vi "TestProgram.vi"() -> ()   [LabVIEW 2011]
uses:
  <instrlib>/Newport ESP301/Newport ESP301.lvlib
panel:
  out "StrehlRatio":dbl=nan
  out "error (scalar)":dbl=nan
  out "Image (IMAQ)":T1(plugin-control)
  in  "Save":bool
  in  "Info":string
  in  "folder":path
  in  "clear daTA":bool
  out "new picture":picture
  out "standard deviation total":dbl=-0.0 format="%0.2f"
  in  "file name":string
  out "Waveform Graph":dbl[][](graph)
  in  "setVelo":dbl=20.0
  in  "cONTINIOUS":bool
  in  "collect daTA":bool
  out "Array":dbl[][](array[numeric])
  out "Value 2":dbl(graph)
  out "Value":dbl(graph)
  out "centroidy":dbl
  out "acceleration":dbl(graph)
  in  "time to wait (TCP) 2":i32=10
  out "Data String":string
  out "shot number":i32=65426
  in  "Device Name":string="StagingFocusBeam2"
  out "centroidx":dbl
  out "Remote Host":string="192.168.10.115"
  out "port or service name":u16=65418
  out "x-y":dbl(knob) scale=0.0..100.0
  out "error out 4":errorcluster
  in  "sTEPsIZE":dbl=5.0
  out "Position (units) 2":dbl(graph)=-13324.641
  in  "ScaN":bool
  in  "shake":bool
  in  "Cluster":T2={"increase"=0.004, "min velocity"=0.1, "max velocity"=3.0, "Stop increase"=0.02}
  out "appended array":dbl[][](graph)=[[1.0, 0.7046880791959296, 0.4965852858533471, 0.3499377259476329, 0.2465969370957652, 0.1737739140097176, 0.12245639698366893, 0.08629355394147512, 0.06081002915927391, 0.0628100291592739, 0.0648100291592739, 0.0668100291592739, 0.06881002915927391, 0.08881002915927391, 0.12881002915927392, 0.18881002915927392, 0.26881002915927393, 0.36881002915927397, 0.48881002915927396, 0.628810029159274, 0.788810029159274, 0.968810029159274, 1.0], [0.0, 0.0, 0.0, 0.0, 0.0, 0.0, 0.004000000000814907, 0.002999999998792191, 0.040000000000873115, 0.20499999999992724, 0.363999999999578, 0.5879999999997381, 0.7160000000003492, 0.7360000000007858, 0.7879999999986467, 0.6760000000012951, 0.3989999999994325, 0.01300000000082946, 0.004000000000814907, 0.003999999998995918, 0.0, 0.0, 0.0], [0.0, 0.0, 0.0, 0.0, 0.0, 0.0, 0.004000000000814907, -0.0010000000020227162, 0.037000000002080924, 0.16499999999905413, 0.15899999999965075, 0.22400000000016007, 0.12800000000061118, 0.020000000000436557, 0.05199999999786087, -0.11199999999735155, -0.27700000000186265, -0.385999999998603, -0.009000000000014552, -1.8189894035458565e-12, -0.003999999998995918, 0.0, 0.0]]
  out "error out 3":errorcluster
  out "ratio":dbl(graph)=1.0
  out "velocity":dbl(graph)
  in  "Velocity (units/s) 2":dbl
  in  "RedRatio":dbl=1.0
  in  "Step":bool
  out "Reduction Ratio":dbl format="%.6g"
  out "Power Status":bool=TRUE
  out "Velocity (units/s)":dbl format="%.4g"
  out "Position (units)":dbl(graph)=-13329.169
  in  "Axis (1)":i32=2
  out "error out":errorcluster
  in  "stop":bool
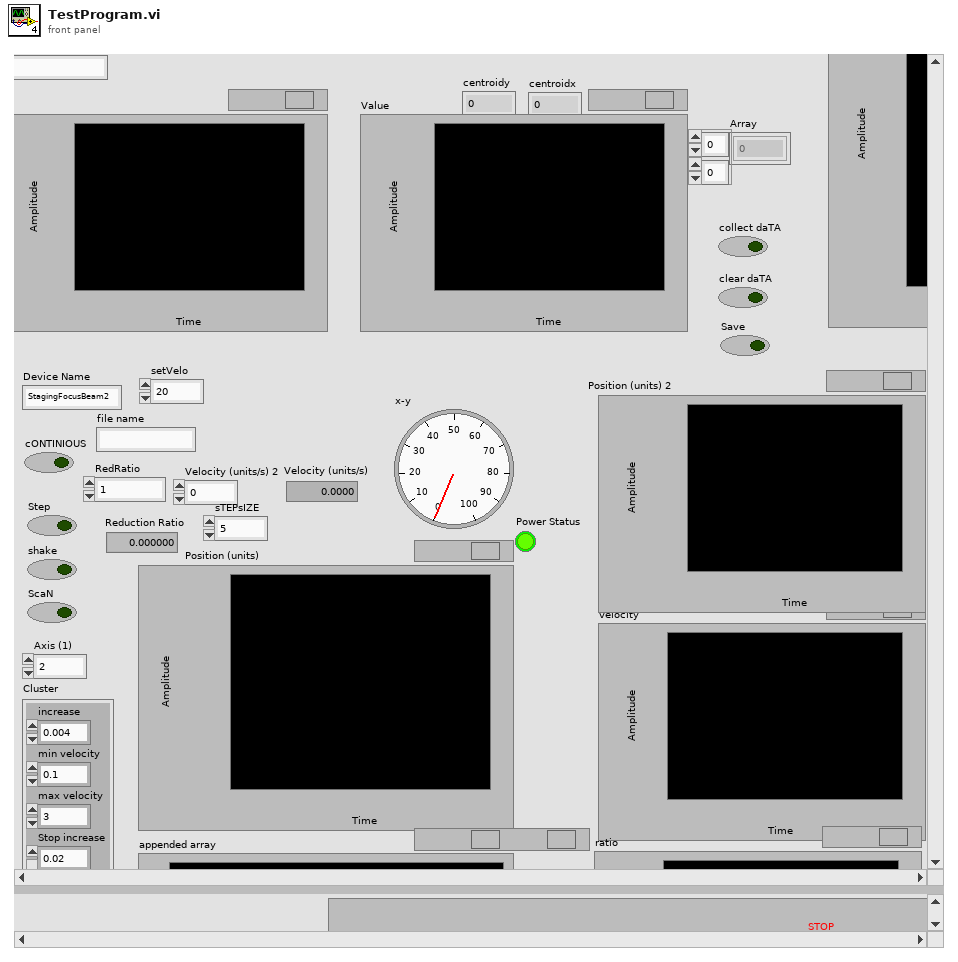
[diagram p1: front panel]
types:
  T1 = typedef "IMAQ Image.ctl" = refnum<image>
  T2 = cluster{"increase":dbl, "min velocity":dbl, "max velocity":dbl, "Stop increase":dbl}
  T3 = typedef "Image Type" = u32
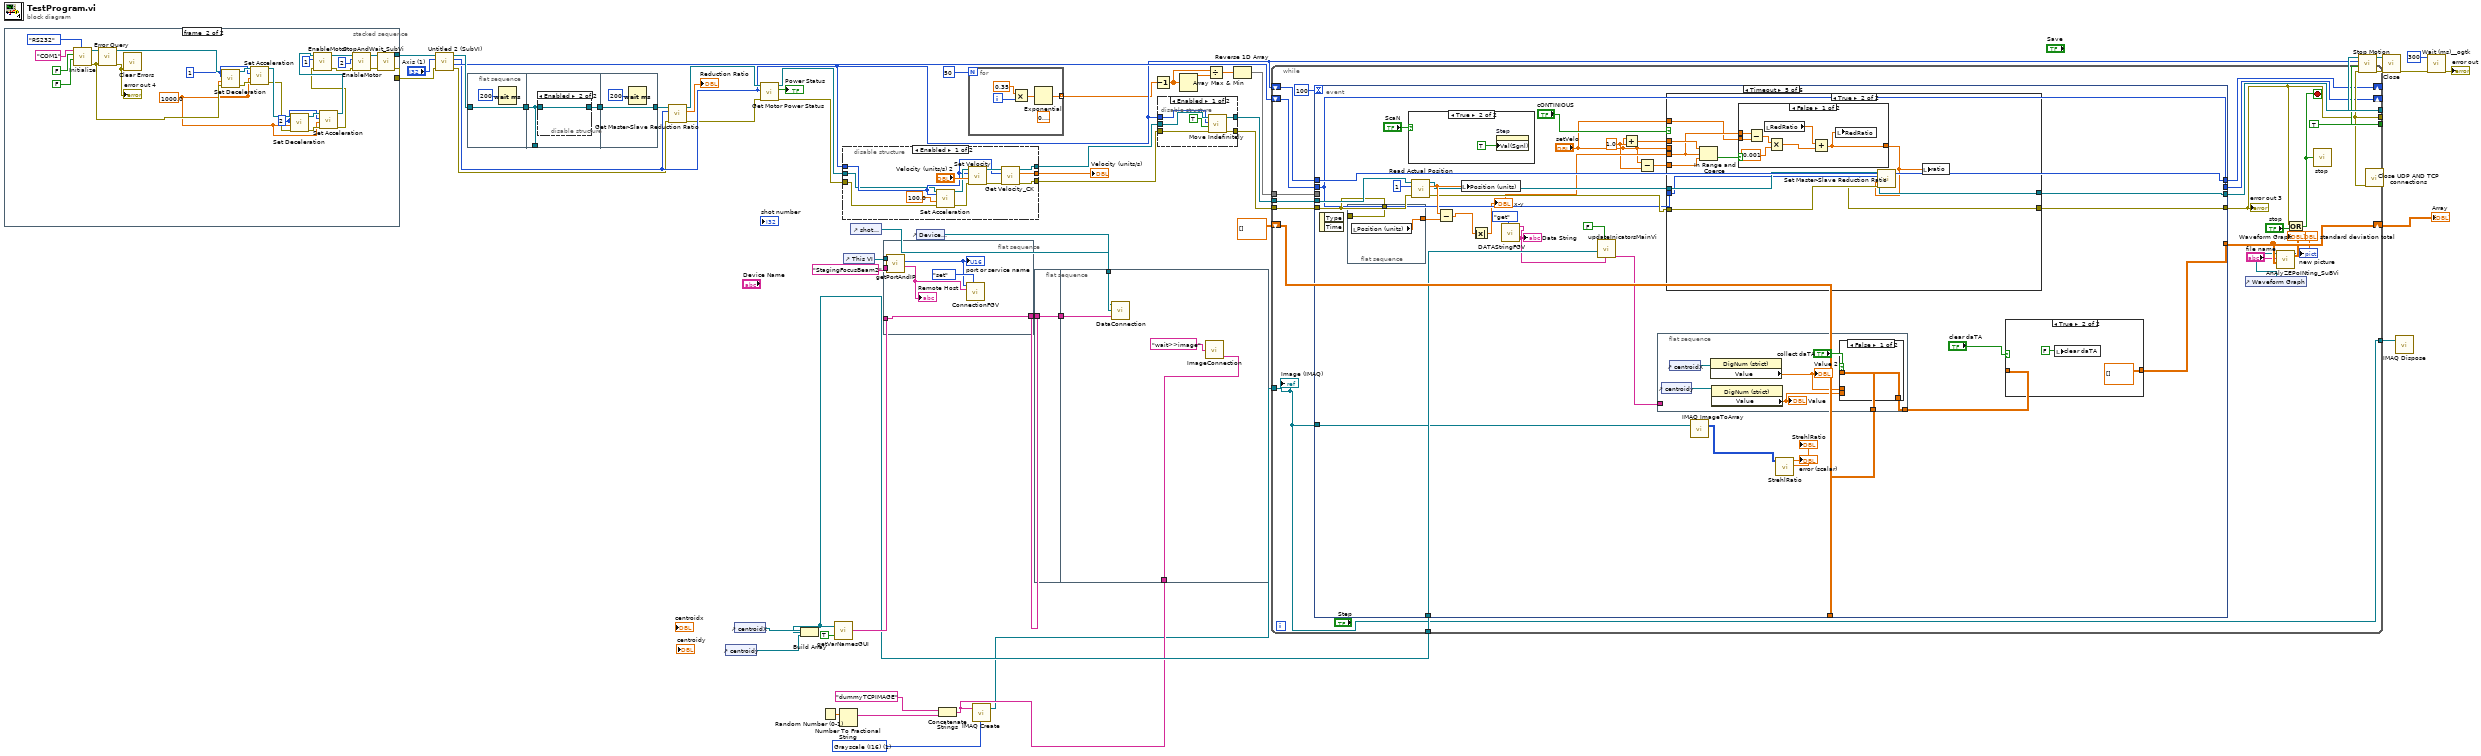
[diagram p0: block diagram]
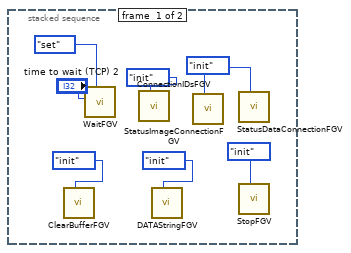
[diagram p2: hidden frame]
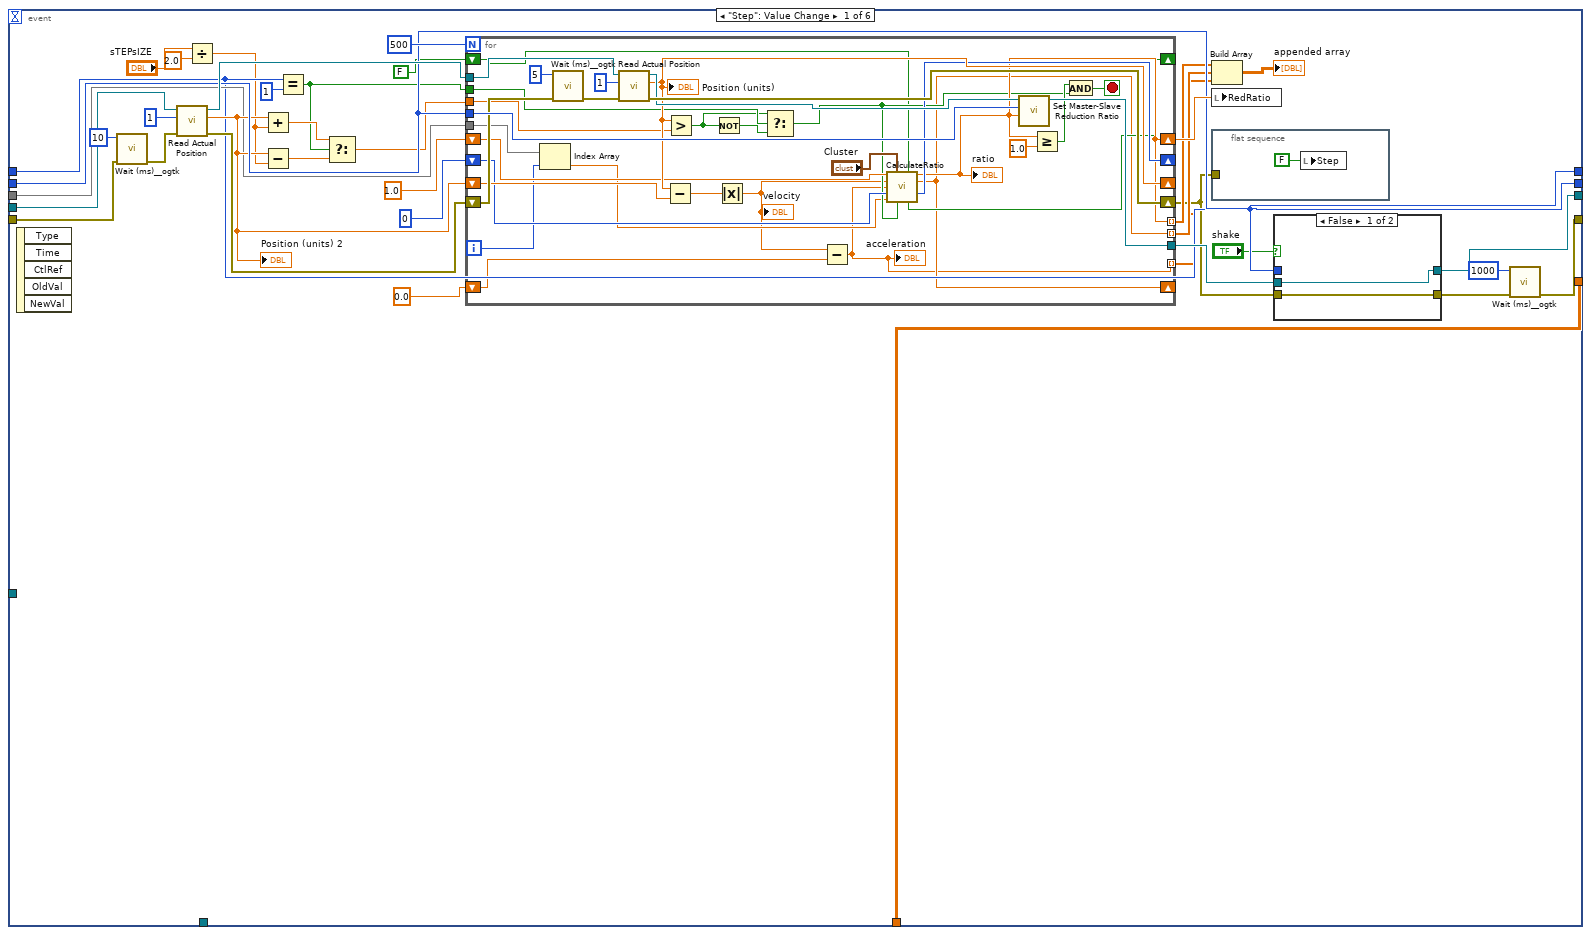
[diagram p3: hidden frame]
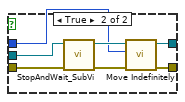
[diagram p4: hidden frame]
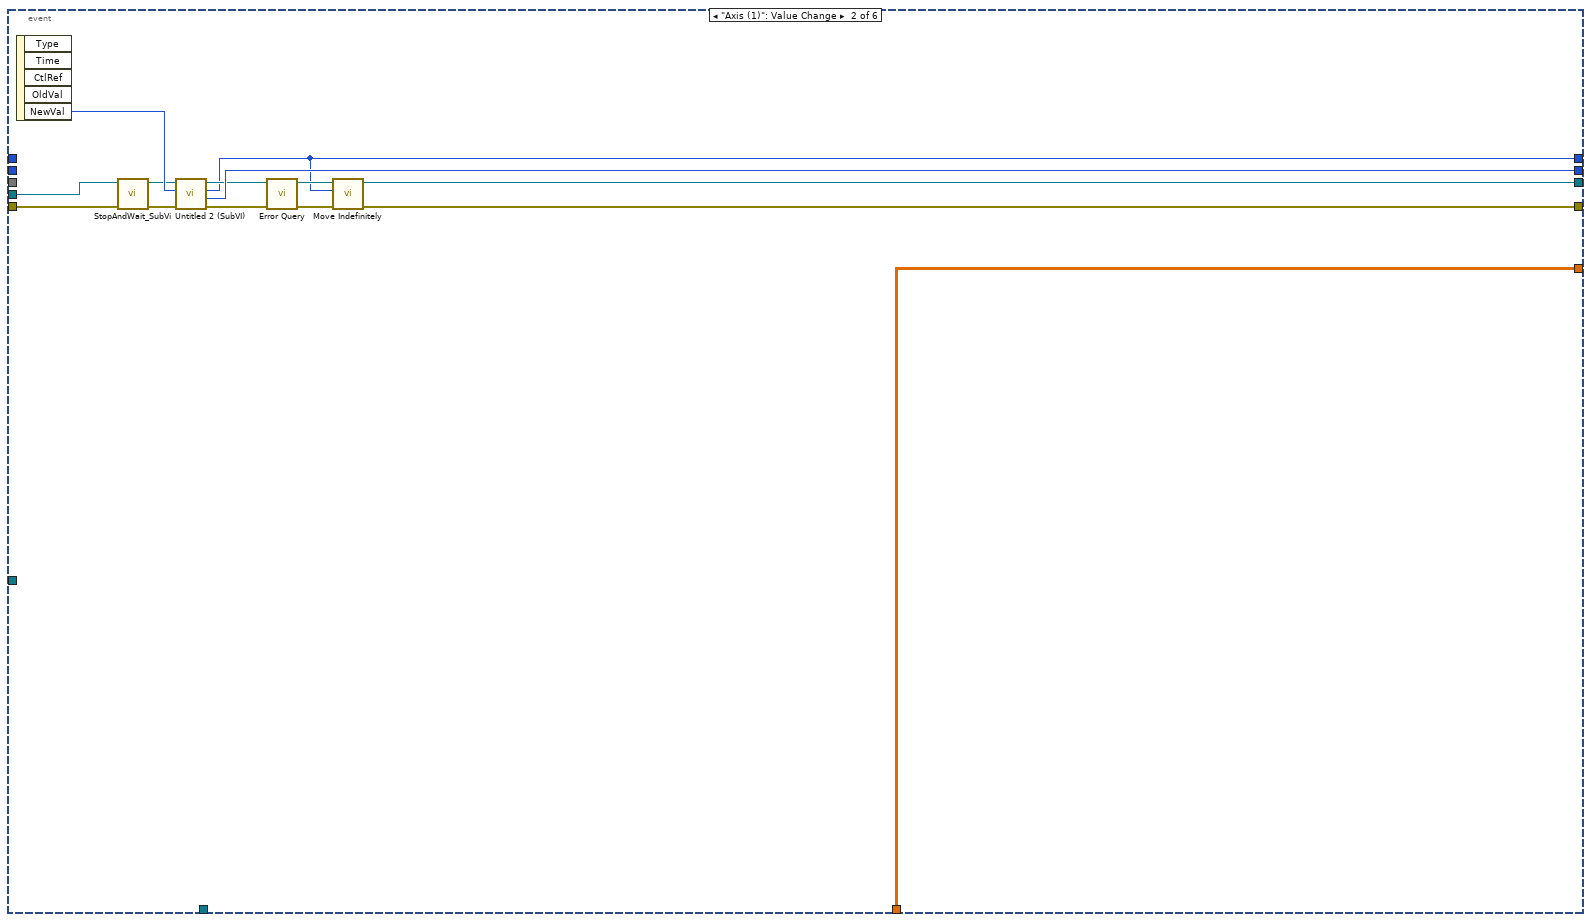
[diagram p5: hidden frame]
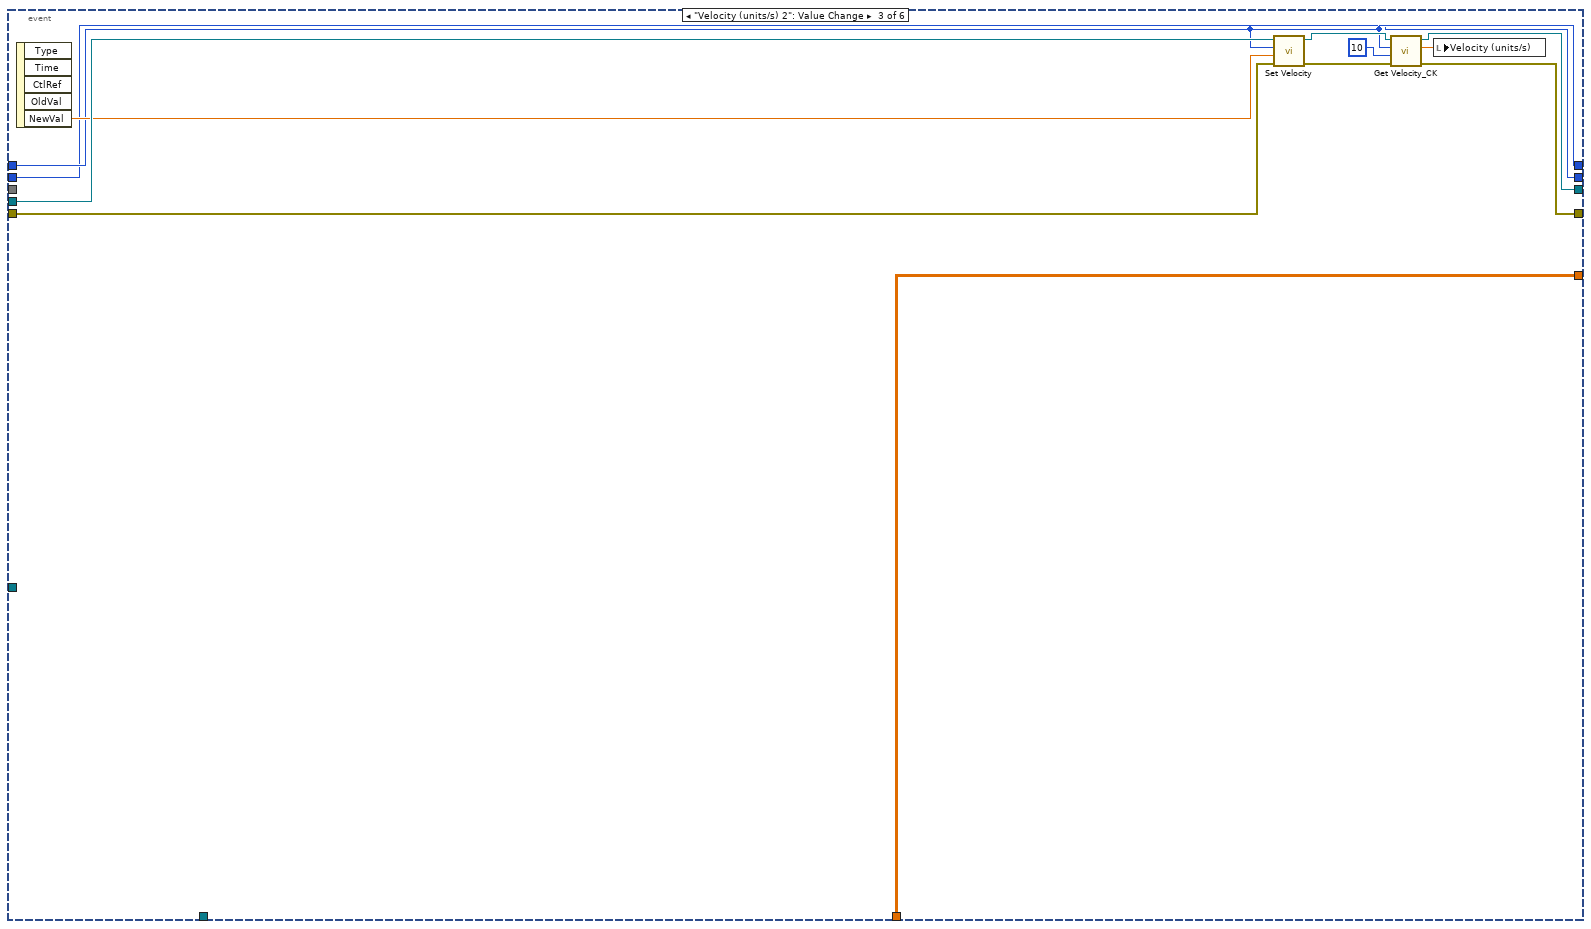
[diagram p6: hidden frame]
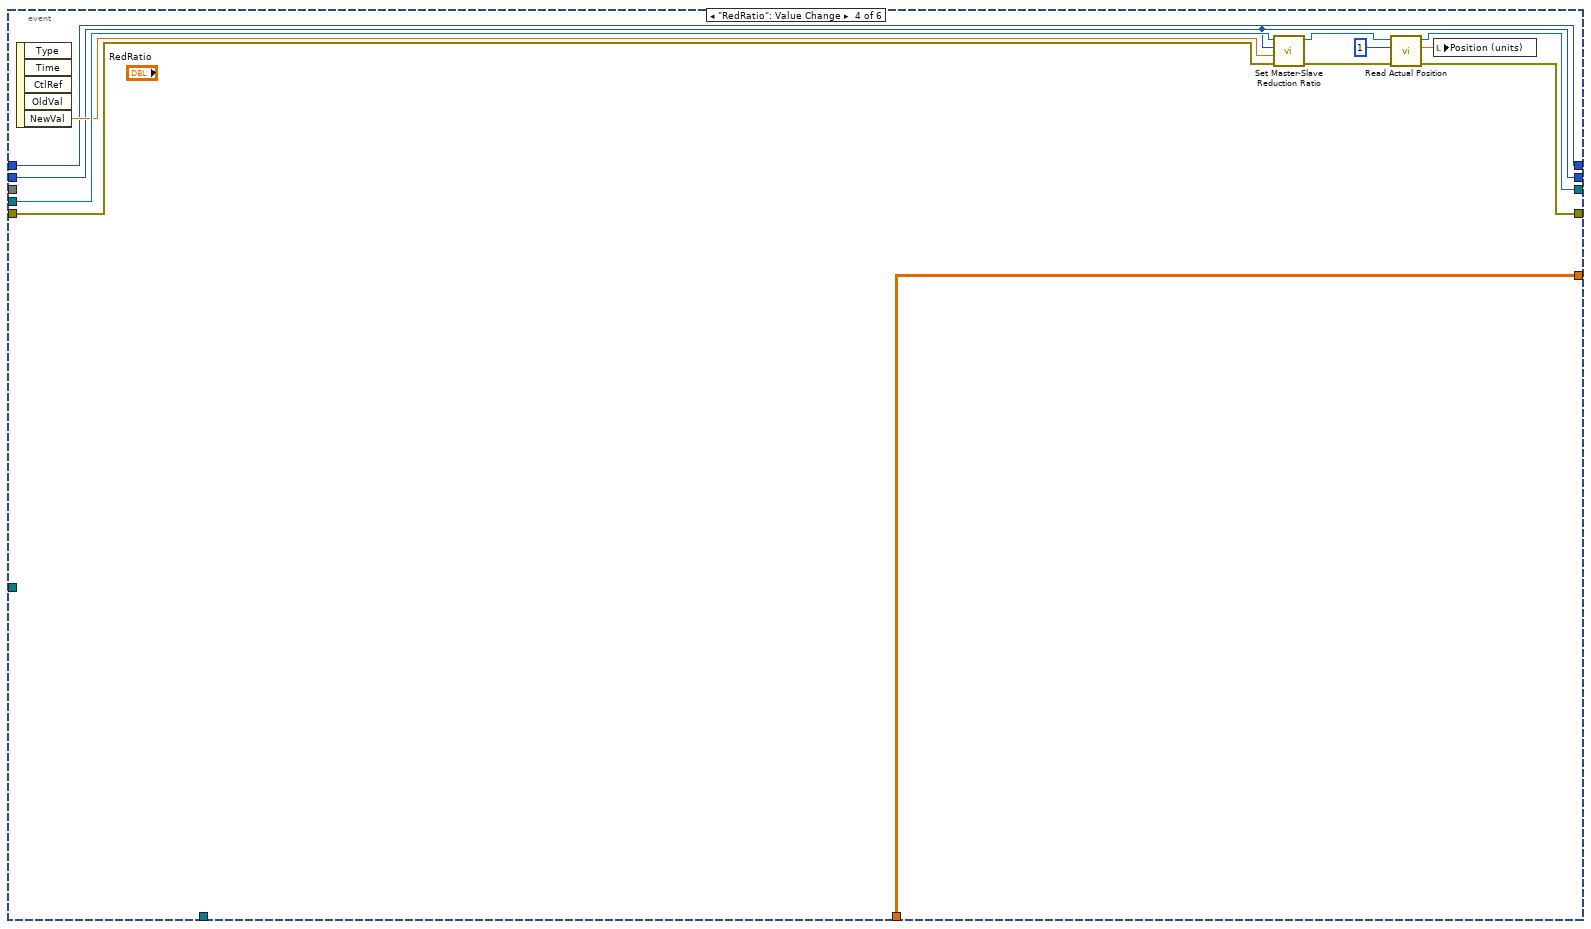
[diagram p7: hidden frame]
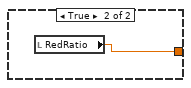
[diagram p10: hidden frame]
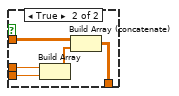
[diagram p11: hidden frame]
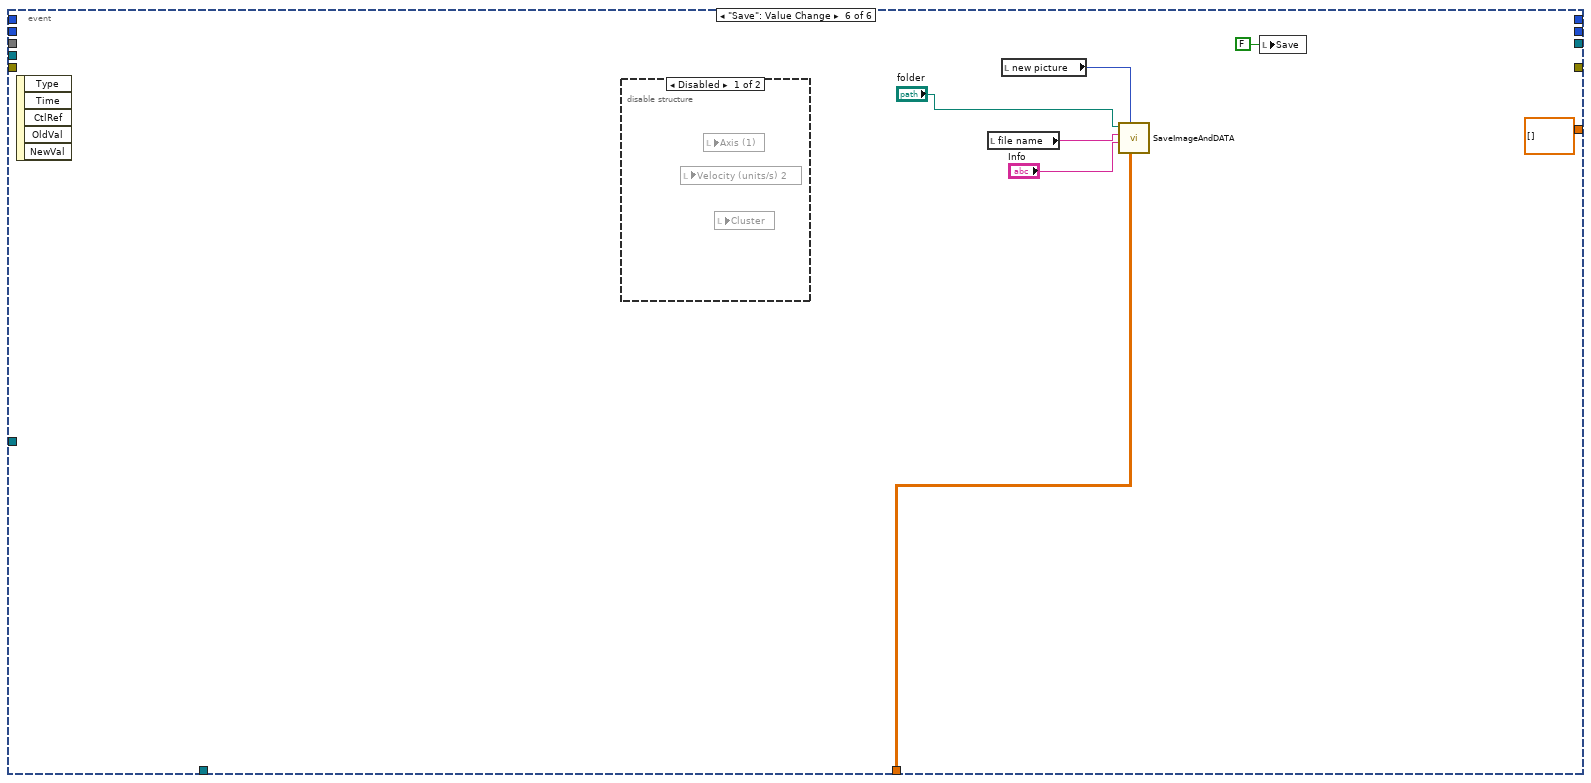
[diagram p13: hidden frame]
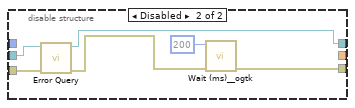
[diagram p15: hidden frame]
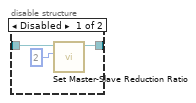
[diagram p16: hidden frame]
diagram:
  w3 = T3 1 items=["Grayscale (U8)", "Grayscale (I16)", "Grayscale (SGL)", "Complex (CSG)", "RGB (U32)", "HSL (U32)", "RGB (U64)", "Grayscale (U16)"] ("Image Type")
  n1 = stacked-sequence {
    tunnel: [_ w85] -> w23
    tunnel: [_ w84] -> w22
    frame #0 {
      w59 = enum16{"get", "set", "init"}."init" ("Command")
      n2 = call "ClearBufferFGV.vi"("Command"=enum16{"set", "get", "init"}."init") -> ()  [unwired: 10 in, 1 out]
      n3 = call "WaitFGV.vi"("Command"=enum16{"get", "set", "init"}."set", "milliseconds to wait"="time to wait (TCP) 2") -> ()  [unwired: 9 in, 1 out]
      n4 = call "ConnectionIDsFGV.vi"("Command"=enum16{"add", "get", "init"}."init") -> ()  [unwired: 10 in, 1 out]
      n5 = call "DATAStringFGV.vi"("Command"=enum16{"get", "set", "init"}."init") -> ()  [unwired: 10 in, 1 out]
      n6 = call "StatusImageConnectionFGV.vi"("Command"=w59) -> ()  [unwired: 10 in, 1 out]
      n7 = call "StatusDataConnectionFGV.vi"("Command"=w59) -> ()  [unwired: 10 in, 1 out]
      n8 = call "StopFGV.vi"("Command"=enum16{"set", "get", "init"}."init") -> ()  [unwired: 10 in, 1 out]
    }
    frame #1 {
      w63 = 2 ("Axis (1)")
      w71 = 1 ("Axis (1) 2")
      w64 = 1000.0 ("Acceleration (0 units/s²)")
      n9 = call <instrlib>:"Initialize.vi"("VISA resource name"="COM1" ("Settings.devport"), "ID Query (True)"=FALSE, "Reset (False)"=FALSE, "Serial Link (RS232)"=enum16{"RS232", "USB"}."RS232") -> ("VISA resource name out"=w83:refnum<visa-resource-name>, "error out"=w73:errorcluster)  [unwired: 5 in]
      n10 = call <instrlib>:"Error Query.vi"("error in (no error)"=w73, "VISA resource name"=w83) -> ("error out"=w82:errorcluster, "VISA resource name out"=w75:refnum<visa-resource-name>)  [unwired: 2 in, 2 out]
      "error out 4" <- w82
      n11 = call <vilib>:"Clear Errors.vi"("error in (no error)"=w82) -> ()  [unwired: 6 in, 1 out]
      n12 = call <instrlib>:"Set Deceleration.vi"("error in (no error)"=w73, "Deceleration (0 units/s²)"=w64, "Axis (1)"=w71, "VISA resource name"=w75) -> ("error out"=w72:errorcluster, "VISA resource name out"=w74:refnum<visa-resource-name>)  [unwired: 2 in]
      n13 = call <instrlib>:"Set Acceleration.vi"("error in (no error)"=w72, "Acceleration (0 units/s²)"=w64, "Axis (1)"=w71, "VISA resource name"=w74) -> ("error out"=w66:errorcluster, "VISA resource name out"=w68:refnum<visa-resource-name>)  [unwired: 2 in]
      n14 = call <instrlib>:"Set Deceleration.vi"("error in (no error)"=w66, "Deceleration (0 units/s²)"=w64, "Axis (1)"=w63, "VISA resource name"=w68) -> ("error out"=w70:errorcluster, "VISA resource name out"=w69:refnum<visa-resource-name>)  [unwired: 2 in]
      n15 = call <instrlib>:"Set Acceleration.vi"("error in (no error)"=w70, "Acceleration (0 units/s²)"=w64, "Axis (1)"=w63, "VISA resource name"=w69) -> ("error out"=w65:errorcluster, "VISA resource name out"=w67:refnum<visa-resource-name>)  [unwired: 2 in]
      n16 = call "EnableMotor.vi"("error in (no error)"=w65, "Axis (1) in"=1, "VISA Refnum in"=w67) -> ("error out"=w79:errorcluster, "VISA Refnum out"=w77:refnum<visa-resource-name>)  [unwired: 7 in]
      n17 = call "EnableMotor.vi"("error in (no error)"=w79, "Axis (1) in"=2, "VISA Refnum in"=w77) -> ("error out"=w78:errorcluster, "VISA Refnum out"=w76:refnum<visa-resource-name>)  [unwired: 7 in]
      n18 = call "StopAndWait_SubVi.vi"("error in (no error)"=w78, "VISA Refnum in"=w76) -> ("error out"=w84:errorcluster, "VISA Refnum out"=w85:refnum<visa-resource-name>)  [unwired: 8 in]
    }
  }
  n19 = call "Untitled 2 (SubVI).vi"("error in (no error)"=w22, "Axis (1)"="Axis (1)", "VISA Refnum in"=w23) -> ("error out"=w26:errorcluster, "Slave"=w35:i32, "Master"=w33:i32, "VISA Refnum out"=w39:refnum<visa-resource-name>)  [unwired: 5 in]
  n20 = flat-sequence {
    tunnel: w39 -> [w91]
    tunnel: [w91] -> w47
    tunnel: [w92] -> _
    tunnel: [w93] -> w48
    tunnel: w47 -> [w92]
    tunnel: [w99] -> w36
    tunnel: w48 -> [w99]
    frame #0 {
      n21 = Wait (ms)(milliseconds to wait=u32 200) -> ()  [unwired: 1 out]
    }
    frame #1 {
      n22 = disable-structure shown="Enabled" {
        disable-tunnel: [w96 w97] -> w93
        disable-tunnel: w92 -> [w94 w97]
        frame Disabled {
          n23 = call <instrlib>:"Set Master-Slave Reduction Ratio.vi"("Axis (1)"=2, "VISA resource name"=w94) -> ("VISA resource name out"=w96:refnum<visa-resource-name>)  [unwired: 4 in, 1 out]
        }
        frame Enabled {
        }
      }
    }
    frame #2 {
      n24 = Wait (ms)(milliseconds to wait=u32 200) -> ()  [unwired: 1 out]
    }
  }
  n25 = call <instrlib>:"Get Master-Slave Reduction Ratio.vi"("error in (no error)"=w26, "Axis (1)"=w33, "VISA resource name"=w36) -> ("error out"=w25:errorcluster, "Reduction Ratio"=→"Reduction Ratio":dbl, "VISA resource name out"=w38:refnum<visa-resource-name>)  [unwired: 2 in]
  n26 = control-ref of="centroidy"() -> (w10:refnum<vi>)
  n27 = control-ref of="centroidX"() -> (w19:refnum<vi>)
  n28 = call <instrlib>:"Get Motor Power Status.vi"("error in (no error)"=w25, "Axis (1)"=w33, "VISA resource name"=w38) -> ("error out"=w24:errorcluster, "Power Status"=→"Power Status":bool, "VISA resource name out"=w44:refnum<visa-resource-name>)  [unwired: 2 in]
  n29 = Build Array(w19, w10) -> (w12:refnum<vi>[])
  n30 = Random Number (0-1)() -> (number: 0 to 1=w4:dbl)
  n31 = call "getVarNamesGUI.vi"("start"=TRUE, "Array"=w12) -> ("String"=w14:string)
  n32 = Number To Fractional String(number=w4) -> (F-format string=w5:string)  [unwired: 3 in]
  n33 = disable-structure shown="Enabled" {
    disable-tunnel: [w111 _] -> w55
    disable-tunnel: [w110 w116] -> w54
    disable-tunnel: w33 -> [w106 _]
    disable-tunnel: w44 -> [w104 w117]
    disable-tunnel: [w100 w113] -> w46
    disable-tunnel: w24 -> [w103 w112]
    frame Enabled {
      n34 = call <instrlib>:"Set Acceleration.vi"("error in (no error)"=w103, "Acceleration (0 units/s²)"=100.0, "Axis (1)"=w106, "VISA resource name"=w104) -> ("error out"=w102:errorcluster, "VISA resource name out"=w107:refnum<visa-resource-name>)  [unwired: 2 in]
      n35 = call <instrlib>:"Set Velocity.vi"("error in (no error)"=w102, "Velocity (units/s)"="Velocity (units/s) 2", "Axis (1)"=w106, "VISA resource name"=w107) -> ("error out"=w101:errorcluster, "VISA resource name out"=w109:refnum<visa-resource-name>)  [unwired: 2 in]
      n36 = call "Get Velocity_CK.vi"("error in (no error)"=w101, "Axis (1)"=w106, "VISA resource name"=w109) -> ("error out"=w100:errorcluster, "Velocity (units/s)"=w111:dbl, "VISA resource name out"=w110:refnum<visa-resource-name>)  [unwired: 2 in]
    }
    frame Disabled {
      n37 = call <instrlib>:"Error Query.vi"("error in (no error)"=w112, "VISA resource name"=w117) -> ("error out"=w115:errorcluster, "VISA resource name out"=w116:refnum<visa-resource-name>)  [unwired: 4 out]
      n38 = call <userlib>:"Wait (ms)__ogtk.vi"("error in (no error)"=w115, "milliseconds to wait"=u32 200) -> ("error out"=w113:errorcluster)  [unwired: 8 in, 1 out]
    }
  }
  "Velocity (units/s)" <- w55
  n39 = control-ref of="This VI"() -> (w21:refnum<vi>)
  n40 = control-ref of="shot number"() -> (w16:refnum<vi>)
  n41 = flat-sequence {
    tunnel: w21 -> [w123]
    tunnel: "StagingFocusBeam2" ("Device Name") -> [w119]
    tunnel: w14 -> [w118]
    tunnel: [w118] -> w13
    frame #0 {
      n42 = call "getPortAndIP.vi"("This Vi"=w123, "Device Name"=w119) -> ("port or service name"=w120:u16, "Remote Host"=w121:string)  [unwired: 1 in, 1 out]
      "port or service name" <- w120
      "Remote Host" <- w121
      n43 = call "ConnectionFGV.vi"("command"=enum16{"get", "set", "init"}."set", "Remote Host in"=w121, "port or service name in"=w120) -> ()  [unwired: 7 in, 2 out]
    }
  }
  n44 = control-ref of="Device Name"() -> (w17:refnum<vi>)
  n45 = Concatenate Strings("dummyTCPIMAGE" ("Image Name"), w5) -> (w2:string)
  n46 = for {
    N: 50 -> [_]
    tunnel: [w127] -> w29 mode=indexing
    i -> [w126]
    (unwired) 0.30000000000000004 ("x")
    n47 = Multiply(x=0.35, y=w126) -> (x*y=w124:dbl)
    n48 = Exponential(1:w124) -> (0:w127:dbl)
  }
  n49 = call "IMAQ Create"("Image Name"=w2, "Image Type"=w3) -> ("New Image"=w1:T1)  [unwired: 3 in, 1 out]
  n50 = flat-sequence {
    tunnel: w13 -> [w128]
    tunnel: [w128] -> w15
    tunnel: w17 -> [w132]
    tunnel: w16 -> [w131]
    tunnel: w15 -> [w133]
    tunnel: w2 -> [w129]
    frame #0 {
    }
    frame #1 {
      n51 = call "DataConnection.vi"("Subscriber list"=w133, "Device Name (h)"=w132, "shotnumber"=w131) -> ()
      n52 = call "ImageConnection.vi"("Image Name"=w129, "Image Subscriber list"="wait>>image") -> ()  [unwired: 2 in]
    }
  }
  n53 = Decrement(x=w29) -> (x-1=w30:dbl[])
  n54 = disable-structure shown="Enabled" {
    disable-tunnel: w54 -> [w139 w140]
    disable-tunnel: [w137 w140] -> w53
    disable-tunnel: w33 -> [w136 _]
    disable-tunnel: w46 -> [w135 _]
    disable-tunnel: [w134 _] -> w45
    frame Enabled {
      n55 = call <instrlib>:"Move Indefinitely.vi"("error in (no error)"=w135, "Move Direction (+)"=TRUE, "Axis (1)"=w136, "VISA resource name"=w139) -> ("error out"=w134:errorcluster, "VISA resource name out"=w137:refnum<visa-resource-name>)  [unwired: 2 in]
    }
    frame Disabled {
    }
  }
  n56 = Array Max & Min(array=w30) -> (max value=w31:dbl)  [unwired: 3 out]
  n57 = Divide(x=w30, y=w31) -> (x/y=w32:dbl[])
  n58 = Reverse 1D Array(array=w32) -> (reversed array=w27:dbl[])
  n59 = while {
    tunnel: w53 -> [w162]
    tunnel: [w161] -> w52
    tunnel: [w156] -> w11
    tunnel: [TRUE ("Stop all axes (F)")] -> w50
    tunnel: w45 -> [w159]
    shift-right: [w153] -> _
    shift-left: w33 -> [w154]
    shift-right: [w152] -> _
    shift-left: w35 -> [w158]
    tunnel: w27 -> [w151]
    tunnel: w12 -> [w150]
    shift-right: [w147] -> w8
    shift-left: dbl[][] [] -> [w148]
    tunnel: w1 -> [w141]
    tunnel: [w141] -> w7
    stop <- w149 stop-if-true
    n60 = event shown="[4] Timeout" {
      selector: _ -> [_ _ _ _ _ _]
      dyn-events: _ -> [_ _ _ _ _ _]
      timeout: 100 -> [_ _ _ _ _ _]
      tunnel: w162 -> [w199 w248 w269 w281 w313 _]
      tunnel: [w179 w249 w265 w275 w297 _] -> w161
      tunnel: w159 -> [w169 w246 w267 w279 w307 _]
      tunnel: w158 -> [w192 _ w259 w271 w294 _]
      tunnel: [w174 w250 w262 w273 w295 _] -> w156
      tunnel: w154 -> [w178 _ w260 w272 w311 _]
      tunnel: [w178 w252 w260 w272 w311 _] -> w153
      tunnel: [w192 w256 w259 w271 w294 _] -> w152
      tunnel: w151 -> [w181 _ _ _ _ _]
      tunnel: w150 -> [_ _ _ _ w305 _]
      tunnel: [w163 w244 w258 w270 w286 dbl[][] []] -> w147
      tunnel: w148 -> [w163 w244 w258 w270 w300 w358]
      tunnel: w141 -> [_ _ _ _ w285 _]
      event "Step": Value Change {
        n61 = event-data() -> ()  [unwired: 1 in, 5 out]
        n62 = call <userlib>:"Wait (ms)__ogtk.vi"("error in (no error)"=w169, "milliseconds to wait"=u32 10) -> ("error out"=w168:errorcluster)  [unwired: 8 in, 1 out]
        n63 = call <instrlib>:"Read Actual Position.vi"("error in (no error)"=w168, "Axis (1)"=1, "VISA resource name"=w199) -> ("error out"=w196:errorcluster, "Position (units)"=w189:dbl, "VISA resource name out"=w198:refnum<visa-resource-name>)  [unwired: 2 in]
        "Position (units) 2" <- w189
        n64 = Divide(x="sTEPsIZE", y=2.0) -> (x/y=w170:dbl)
        n65 = Add(x=w189, y=w170) -> (x+y=w190:dbl)
        n66 = Subtract(x=w189, y=w170) -> (x-y=w188:dbl)
        n67 = Equal?(x=w178, y=1) -> (x = y?=w186:bool)
        n68 = Select(t=w190, s=w186, f=w188) -> (s? t:f=w187:dbl)
        n69 = for {
          N: 500 -> [_]
          tunnel: [w239] -> w180
          tunnel: w198 -> [w241]
          shift-right: [w242] -> w176
          shift-left: w196 -> [w237]
          tunnel: w192 -> [w238]
          shift-right: [w232] -> _
          shift-left: w189 -> [w234]
          shift-right: [w224] -> w193
          shift-left: 1.0 -> [w223]
          tunnel: w187 -> [w231]
          tunnel: w186 -> [w229]
          shift-right: [w225] -> _
          shift-left: 0 -> [w226]
          tunnel: [w224] -> w184 mode=indexing
          tunnel: [w211] -> w183 mode=indexing
          tunnel: w181 -> [w216]
          shift-right: [w217] -> _
          shift-left: FALSE -> [w218]
          shift-right: [w211] -> _
          shift-left: 0.0 -> [w212]
          tunnel: [w210] -> w164 mode=indexing
          i -> [w215]
          stop <- w219 stop-if-true
          n70 = Index Array(array=w216, index=w215) -> (element=w214:dbl)
          n71 = call <userlib>:"Wait (ms)__ogtk.vi"("error in (no error)"=w237, "milliseconds to wait"=u32 5) -> ("error out"=w236:errorcluster)  [unwired: 8 in, 1 out]
          n72 = call <instrlib>:"Read Actual Position.vi"("error in (no error)"=w236, "Axis (1)"=1, "VISA resource name"=w241) -> ("error out"=w242:errorcluster, "Position (units)"=w232:dbl, "VISA resource name out"=w240:refnum<visa-resource-name>)  [unwired: 2 in]
          "Position (units)" <- w232
          n73 = Subtract(x=w232, y=w234) -> (x-y=w233:dbl)
          n74 = Greater?(x=w232, y=w231) -> (0:w227:bool)
          n75 = Not(x=w227) -> (.not. x?=w228:bool)
          n76 = Absolute Value(x=w233) -> (abs(x)=w213:dbl)
          "velocity" <- w213
          n77 = Select(t=w227, s=w229, f=w228) -> (s? t:f=w220:bool)
          n78 = Subtract(x=w213, y=w212) -> (x-y=w210:dbl)
          "acceleration" <- w210
          n79 = call "CalculateRatio.vi"("ratio"=w223, "Cluster"="Cluster", "decrease again"=w218, "velocity"=w213, "acceleration"=w210, "rep"=w226, "downramp"=w214, "stop"=w220) -> ("ratio out"=w224:dbl, "velocity out"=w211:dbl, "rep out"=w225:i32, "decrease again out"=w217:bool)  [unwired: 4 in]
          "ratio" <- w224
          n80 = call <instrlib>:"Set Master-Slave Reduction Ratio.vi"("Reduction Ratio (0)"=w224, "Axis (1)"=w238, "VISA resource name"=w240) -> ("VISA resource name out"=w239:refnum<visa-resource-name>)  [unwired: 3 in, 1 out]
          n81 = Greater Or Equal?(x=w224, y=1.0) -> (x >= y?=w221:bool)
          n82 = And(x=w221, y=w220) -> (x .and. y?=w219:bool)
        }
        n83 = Build Array(w184, w183, w164) -> (→"appended array":dbl[][])
        n84 = local write "RedRatio"(w193) -> ()
        n85 = flat-sequence {
          tunnel: w176 -> [_]
          frame #0 {
            n86 = local write "Step"(FALSE ("Step")) -> ()
          }
        }
        n87 = case shown="False" "shake" {
          tunnel: w180 -> [w201 w208]
          tunnel: [w201 w206] -> w179
          tunnel: w178 -> [_ w205]
          tunnel: w176 -> [w200 w204]
          tunnel: [w200 w202] -> w175
          frame False {
          }
          frame True {
            n88 = call "StopAndWait_SubVi.vi"("error in (no error)"=w204, "VISA Refnum in"=w208) -> ("error out"=w203:errorcluster, "VISA Refnum out"=w207:refnum<visa-resource-name>)  [unwired: 8 in]
            n89 = call <instrlib>:"Move Indefinitely.vi"("error in (no error)"=w203, "Axis (1)"=w205, "VISA resource name"=w207) -> ("error out"=w202:errorcluster, "VISA resource name out"=w206:refnum<visa-resource-name>)  [unwired: 3 in]
          }
        }
        n90 = call <userlib>:"Wait (ms)__ogtk.vi"("error in (no error)"=w175, "milliseconds to wait"=u32 1000) -> ("error out"=w174:errorcluster)  [unwired: 8 in, 1 out]
      }
      event "Axis (1)": Value Change {
        n91 = event-data() -> ("NewVal"=w257:i32)  [unwired: 1 in, 4 out]
        n92 = call "StopAndWait_SubVi.vi"("error in (no error)"=w246, "VISA Refnum in"=w248) -> ("error out"=w245:errorcluster, "VISA Refnum out"=w247:refnum<visa-resource-name>)  [unwired: 8 in]
        n93 = call "Untitled 2 (SubVI).vi"("error in (no error)"=w245, "Axis (1)"=w257, "VISA Refnum in"=w247) -> ("error out"=w254:errorcluster, "Slave"=w256:i32, "Master"=w252:i32, "VISA Refnum out"=w255:refnum<visa-resource-name>)  [unwired: 5 in]
        n94 = call <instrlib>:"Error Query.vi"("error in (no error)"=w254, "VISA resource name"=w255) -> ("error out"=w251:errorcluster, "VISA resource name out"=w253:refnum<visa-resource-name>)  [unwired: 2 in, 2 out]
        n95 = call <instrlib>:"Move Indefinitely.vi"("error in (no error)"=w251, "Axis (1)"=w252, "VISA resource name"=w253) -> ("error out"=w250:errorcluster, "VISA resource name out"=w249:refnum<visa-resource-name>)  [unwired: 3 in]
      }
      event "Velocity (units/s) 2": Value Change {
        n96 = event-data() -> ("NewVal"=w268:dbl)  [unwired: 1 in, 4 out]
        n97 = call <instrlib>:"Set Velocity.vi"("error in (no error)"=w267, "Velocity (units/s)"=w268, "Axis (1)"=w260, "VISA resource name"=w269) -> ("error out"=w263:errorcluster, "VISA resource name out"=w266:refnum<visa-resource-name>)  [unwired: 2 in]
        n98 = call "Get Velocity_CK.vi"("error in (no error)"=w263, "Wait before read (0ms)"=u32 10, "Axis (1)"=w260, "VISA resource name"=w266) -> ("error out"=w262:errorcluster, "Velocity (units/s)"=w261:dbl, "VISA resource name out"=w265:refnum<visa-resource-name>)  [unwired: 1 in]
        n99 = local write "Velocity (units/s)"(w261) -> ()
      }
      event "RedRatio": Value Change {
        n100 = event-data() -> ("NewVal"=w280:dbl)  [unwired: 1 in, 4 out]
        n101 = call <instrlib>:"Set Master-Slave Reduction Ratio.vi"("error in (no error)"=w279, "Reduction Ratio (0)"=w280, "Axis (1)"=w271, "VISA resource name"=w281) -> ("error out"=w274:errorcluster, "VISA resource name out"=w276:refnum<visa-resource-name>)  [unwired: 2 in]
        n102 = call <instrlib>:"Read Actual Position.vi"("error in (no error)"=w274, "Axis (1)"=1, "VISA resource name"=w276) -> ("error out"=w273:errorcluster, "Position (units)"=w278:dbl, "VISA resource name out"=w275:refnum<visa-resource-name>)  [unwired: 2 in]
        n103 = local write "Position (units)"(w278) -> ()
      }
      event Timeout {
        w292 = 1.0 ("y")
        n104 = event-data() -> ()  [unwired: 1 in, 2 out]
        n105 = flat-sequence {
          tunnel: [w352] -> w308
          tunnel: [w351] -> _
          tunnel: w307 -> [w351]
          frame #0 {
            n106 = local read "Position (units)"() -> (w352:dbl)
          }
        }
        n107 = case shown="True" "ScaN" {
          frame False {
          }
          frame True {
            n108 = property on="Step" class="Bool (strict)"("Val(Sgnl)"=TRUE ("Value (Signaling)")) -> ()  [unwired: 2 in, 2 out]
          }
        }
        n109 = call <instrlib>:"Read Actual Position.vi"("error in (no error)"=w307, "Axis (1)"=1, "VISA resource name"=w313) -> ("error out"=w296:errorcluster, "Position (units)"=w309:dbl, "VISA resource name out"=w298:refnum<visa-resource-name>)  [unwired: 2 in]
        n110 = Subtract(x=w309, y=w308) -> (x-y=w306:dbl)
        n111 = local write "Position (units)"(w309) -> ()
        n112 = Absolute Value(x=w306) -> (abs(x)=w293:dbl)
        "x-y" <- w293
        n113 = call "DATAStringFGV.vi"("Command"=enum16{"get", "set", "init"}."get") -> ("Data String out"=w303:string)  [unwired: 10 in]
        "Data String" <- w303
        n114 = call "updateInicatorsMainVi.vi"("Data String out"=w303, "Boolean"=FALSE, "Array"=w305) -> ("Data String out 2"=w301:string)  [unwired: 6 in, 2 out]
        n115 = Add(x="setVelo", y=w292) -> (x+y=w291:dbl)
        n116 = Subtract(x="setVelo", y=w292) -> (x-y=w290:dbl)
        n117 = flat-sequence {
          tunnel: w301 -> [_]
          tunnel: [w340] -> w288
          tunnel: w300 -> [w339]
          frame #0 {
            n118 = control-ref of="centroidy"() -> (w343:refnum<vi>)
            n119 = control-ref of="centroidX"() -> (w344:refnum<vi>)
            n120 = property class="DigNum (strict)"(reference=w344) -> ("Value"=w342:dbl)  [unwired: 1 in, 2 out]
            "Value 2" <- w342
            n121 = property class="DigNum (strict)"(reference=w343) -> ("Value"=w341:dbl)  [unwired: 1 in, 2 out]
            "Value" <- w341
            n122 = case shown="False" "collect daTA" {
              tunnel: w342 -> [_ w350]
              tunnel: w341 -> [_ w349]
              tunnel: [w345 w347] -> w340
              tunnel: w339 -> [w345 w346]
              frame False {
              }
              frame True {
                n123 = Build Array(w350, w349) -> (w348:dbl[])
                n124 = Build Array (concatenate)(w346, w348) -> (w347:dbl[][])
              }
            }
          }
        }
        n125 = case shown="True" "cONTINIOUS" {
          tunnel: w298 -> [w318 w329]
          tunnel: [w318 w328] -> w297
          tunnel: w296 -> [w317 w327]
          tunnel: [w317 w326] -> w295
          tunnel: w294 -> [_ w325]
          tunnel: "setVelo" -> [_ _]
          tunnel: w293 -> [_ w321]
          tunnel: w291 -> [_ w324]
          tunnel: w290 -> [_ w323]
          tunnel: "setVelo" -> [_ w320]
          frame False {
          }
          frame True {
            n126 = In Range and Coerce(upper limit=w324, x=w321, lower limit=w323) -> (In Range?=w322:bool)  [unwired: 1 out]
            n127 = case shown="False" w322 {
              tunnel: w321 -> [w335 _]
              tunnel: w320 -> [w334 _]
              tunnel: [w330 w337] -> w319
              frame False {
                n128 = Subtract(x=w335, y=w334) -> (x-y=w333:dbl)
                n129 = local read "RedRatio"() -> (w336:dbl)
                n130 = Multiply(x=w333, y=0.001) -> (x*y=w331:dbl)
                n131 = Add(x=w336, y=w331) -> (x+y=w330:dbl)
                n132 = local write "RedRatio"(w330) -> ()
              }
              frame True {
                n133 = local read "RedRatio"() -> (w337:dbl)
              }
            }
            n134 = call <instrlib>:"Set Master-Slave Reduction Ratio.vi"("error in (no error)"=w327, "Reduction Ratio (0)"=w319, "Axis (1)"=w325, "VISA resource name"=w329) -> ("error out"=w326:errorcluster, "VISA resource name out"=w328:refnum<visa-resource-name>)  [unwired: 2 in]
            n135 = local write "ratio"(w319) -> ()
          }
        }
        n136 = call "IMAQ ImageToArray"("Image"=w285) -> ("Image Pixels (U8)"=w284:u8[][])  [unwired: 3 in, 4 out]
        n137 = call "StrehlRatio.vi"("Image Pixels (I16)"=w284) -> ("StrehlRatio"=→"StrehlRatio":dbl, "error (scalar)"=→"error (scalar)":dbl)  [unwired: 7 in, 2 out]
        n138 = case shown="True" "clear daTA" {
          tunnel: w288 -> [w314 _]
          tunnel: [w314 dbl[][] []] -> w286
          frame False {
          }
          frame True {
            n139 = local write "clear daTA"(FALSE ("clear daTA")) -> ()
          }
        }
      }
      event "Save": Value Change {
        n140 = event-data() -> ()  [unwired: 1 in, 5 out]
        n141 = disable-structure shown="Disabled" {
          frame Disabled {
            n142 = local read "Velocity (units/s) 2"() -> ()  [unwired: 1 in]
            n143 = local read "Axis (1)"() -> ()  [unwired: 1 in]
            n144 = local read "Cluster"() -> ()  [unwired: 1 in]
          }
          frame Enabled {
          }
        }
        n145 = local read "file name"() -> (w360:string)
        n146 = local read "new picture"() -> (w359:picture)
        n147 = call "SaveImageAndDATA.vi"("Array"=w358, "new picture"=w359, "Info"="Info", "file name"=w360, "folder"="folder") -> ()  [unwired: 7 in]
        n148 = local write "Save"(FALSE ("Save")) -> ()
      }
    }
    "error out 3" <- w156
    n149 = control-ref of="Waveform Graph"() -> (w145:refnum<vi>)
    n150 = call "AnAlyZEPoINting_SuBVi.vi"("Array in"=w147, "file name"="file name", "WaveformGraph in"=w145) -> ("new picture"=→"new picture":picture, "standard deviation total"=→"standard deviation total":dbl, "Waveform Graph"=→"Waveform Graph":dbl[][])  [unwired: 2 in, 4 out]
    n151 = Or(x=w156, y="stop") -> (x .or. y?=w149:bool)
    n152 = call "stop.vi"("Boolean"=w149) -> ()
    "Image (IMAQ)" <- w141
  }
  "Array" <- w8
  n153 = call <instrlib>:"Stop Motion.vi"("error in (no error)"=w11, "Stop all axes (F)"=w50, "Axis (1)"=w33, "VISA resource name"=w52) -> ("error out"=w49:errorcluster, "VISA resource name out"=w51:refnum<visa-resource-name>)  [unwired: 2 in]
  n154 = call "Close UDP AND TCP connections.vi"("error in"=w11) -> ()  [unwired: 7 in]
  n155 = call <instrlib>:"Close.vi"("error in (no error)"=w49, "VISA resource name"=w51) -> ("error out"=w42:errorcluster)  [unwired: 9 in]
  n156 = call "IMAQ Dispose"("Image"=w7) -> ()  [unwired: 5 in, 1 out]
  n157 = call <userlib>:"Wait (ms)__ogtk.vi"("error in (no error)"=w42, "milliseconds to wait"=u32 300) -> ("error out"=→"error out":errorcluster)  [unwired: 8 in, 1 out]
